vi "运行时菜单3.vi"   [LabVIEW 2018]
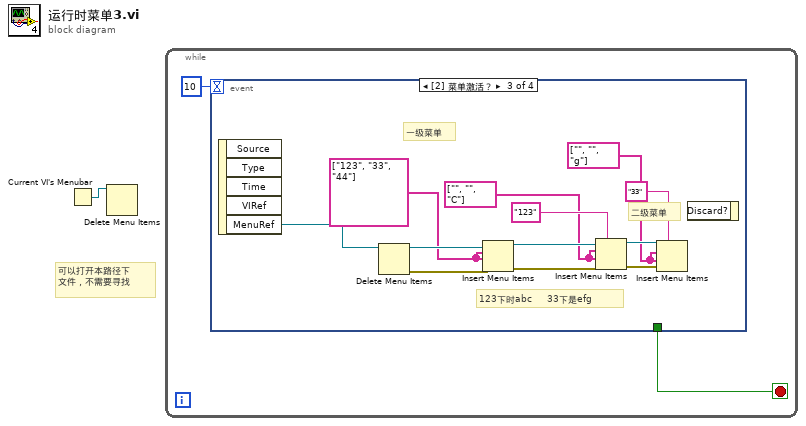
[diagram p0: block diagram]
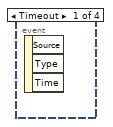
[diagram p2: hidden frame]
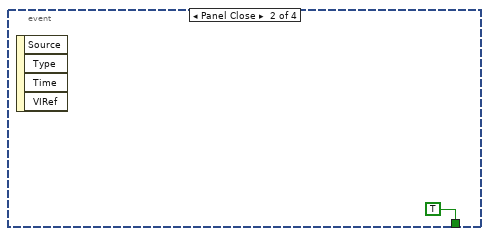
[diagram p3: hidden frame]
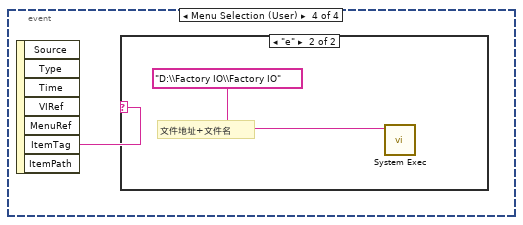
[diagram p4: hidden frame]
diagram:
  # "可以打开本路径下\n文件，不需要寻找"
  n1 = Current VI's Menubar() -> (w1:refnum<k9>)
  n2 = Delete Menu Items(9:w1) -> ()  [unwired: 3 in, 2 out]
  n3 = while {
    stop <- w2 stop-if-true
    n4 = event shown="[2] 菜单激活？" {
      selector: _ -> [_ _ _ _]
      dyn-events: _ -> [_ _ _ _]
      timeout: 10 -> [_ _ _ _]
      tunnel: [_ TRUE ("停止") _ _] -> w2
      event Timeout {
        n5 = event-data() -> ()  [unwired: 1 in, 3 out]
      }
      event Panel Close {
        n6 = event-data() -> ()  [unwired: 1 in, 4 out]
      }
      event Menu Activation? {
        w6 = string[] ["", "", "g"] ("项标识符")
        w9 = string[] ["", "", "C"] ("项标识符")
        w14 = string[] ["123", "33", "44"] ("项标识符")
        # "123下时abc     33下是efg"
        # "二级菜单"
        # "一级菜单"
        n7 = event-data() -> ("MenuRef"=w16:refnum<k9>)  [unwired: 1 in, 4 out]
        n8 = Delete Menu Items(9:w16) -> (0:w13:errorcluster, 3:w15:refnum<k9>)  [unwired: 3 in]
        n9 = Insert Menu Items(6:w13, 7:w14, 8:w14, 9:w15) -> (0:w11:errorcluster, 3:w12:refnum<k9>)  [unwired: 2 in, 1 out]
        n10 = Insert Menu Items(5:"123" ("菜单标识符"), 6:w11, 7:w9, 8:w9, 9:w12) -> (0:w7:errorcluster, 3:w8:refnum<k9>)  [unwired: 1 in, 1 out]
        n11 = Insert Menu Items(5:"33" ("菜单标识符"), 6:w7, 7:w6, 8:w6, 9:w8) -> ()  [unwired: 1 in, 3 out]
        n12 = event-data() -> ()  [unwired: 2 in, 1 out]
      }
      event Menu Selection (User) {
        n13 = event-data() -> ("ItemTag"=w17:string)  [unwired: 1 in, 6 out]
        n14 = case shown="\"e\"" w17 {
          frame "假", Default {
          }
          frame "e" {
            # "文件地址+文件名"
            n15 = call <vilib>:"System Exec.vi"("command line"="D:\\Factory IO\\Factory IO") -> ()  [unwired: 7 in, 4 out]
          }
        }
      }
    }
  }
